vi "SEQUENCE_subVI_V2.vi"(0 "current step # in":i32, 5 "user sequence in":dbl[][](array[numeric]), 9 "input data":T1) -> (2 "pressure control settings out":T2, 3 "sequence on?":bool, 4 "vapor and gas flow out":dbl[](array[numeric]), 6 "sequence end time":timestamp, 10 "current  step # out":i32, 12 "time spent running":dbl)   [LabVIEW 2014]
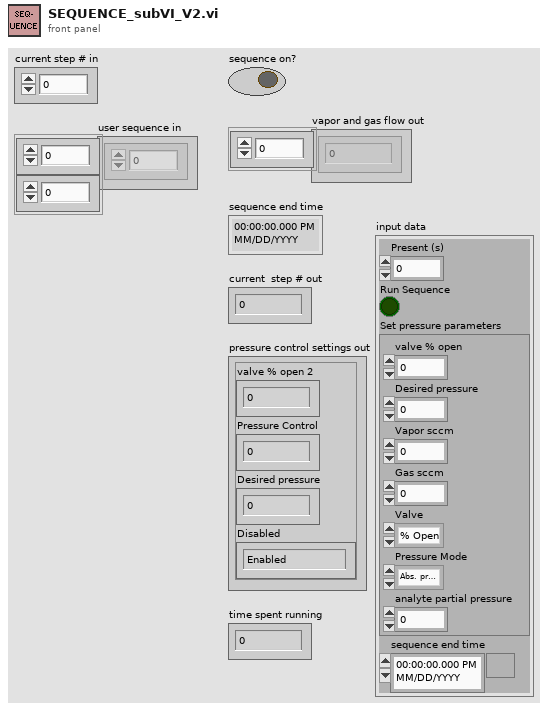
[diagram p1: front panel]
types:
  T1 = cluster{"Present (s)":dbl, "Run Sequence":bool, "Set pressure parameters":cluster{"valve % open":dbl, "Desired pressure":dbl, "Vapor sccm":sgl, "Gas sccm":sgl, "Valve":enum32{"% Open", "Torr "}, "Pressure Mode":enum32{"Abs. pressure", " Part. pressure"}, "analyte partial pressure":dbl}, "sequence end time":timestamp}
  T2 = cluster{"valve % open 2":dbl, "Pressure Control":u32, "Desired pressure":dbl, "Disabled":enum8{"Enabled", "Disabled", "Disabled and Grayed Out"}}
  T3 = cluster{"valve % open":dbl, "Desired pressure":dbl, "Vapor sccm":sgl, "Gas sccm":sgl, "Valve":enum32{"% Open", "Torr "}, "Pressure Mode":enum32{"Abs. pressure", " Part. pressure"}, "analyte partial pressure":dbl}
  T4 = enum8{"Enabled", "Disabled", "Disabled and Grayed Out"}
  T5 = cluster{"valve % open 2":dbl, "Pressure Control":u32, "Numeric Control":dbl, "Disabled":enum8{"Enabled", "Disabled", "Disabled and Grayed Out"}}
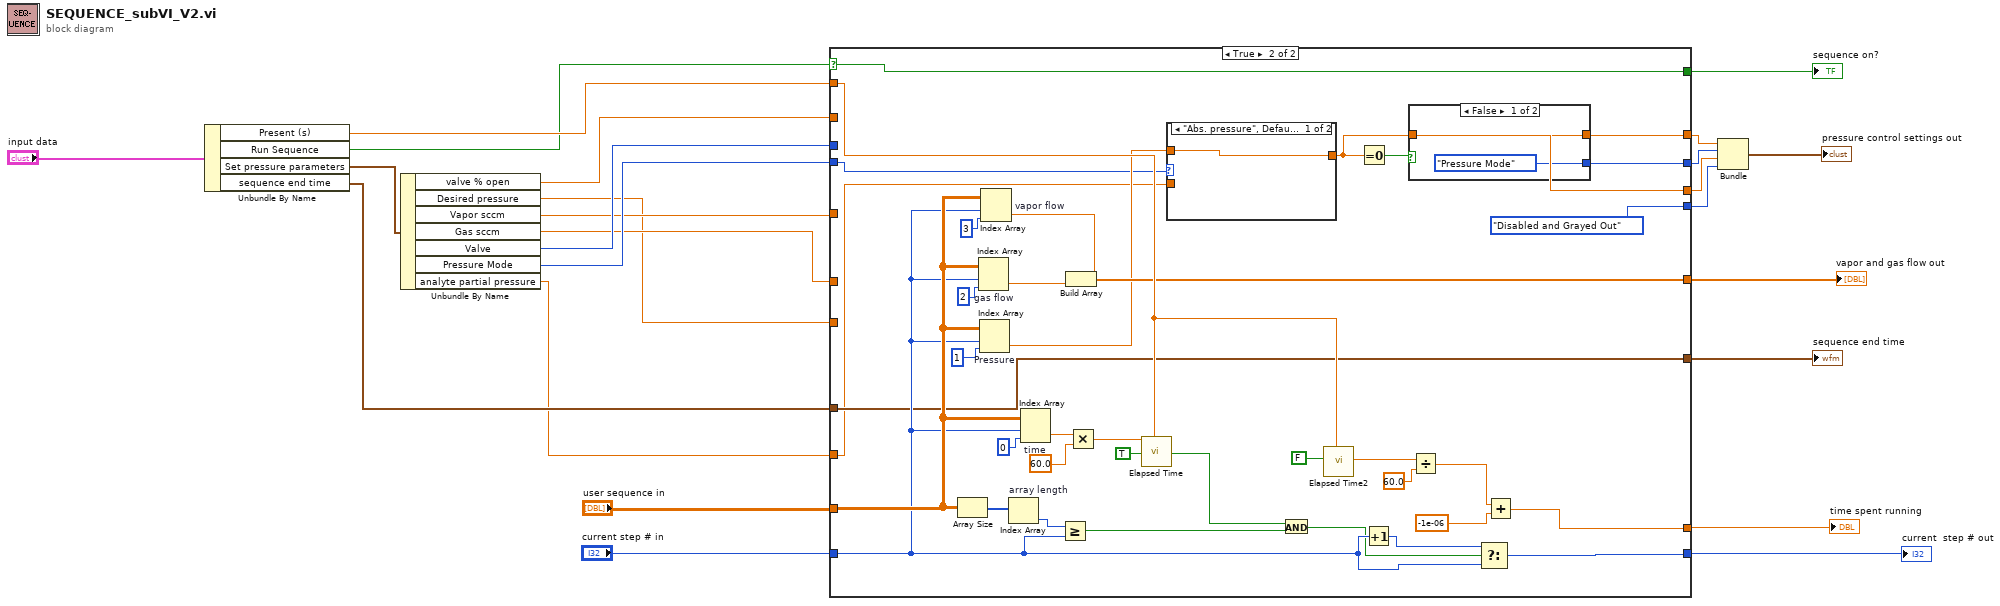
[diagram p0: block diagram]
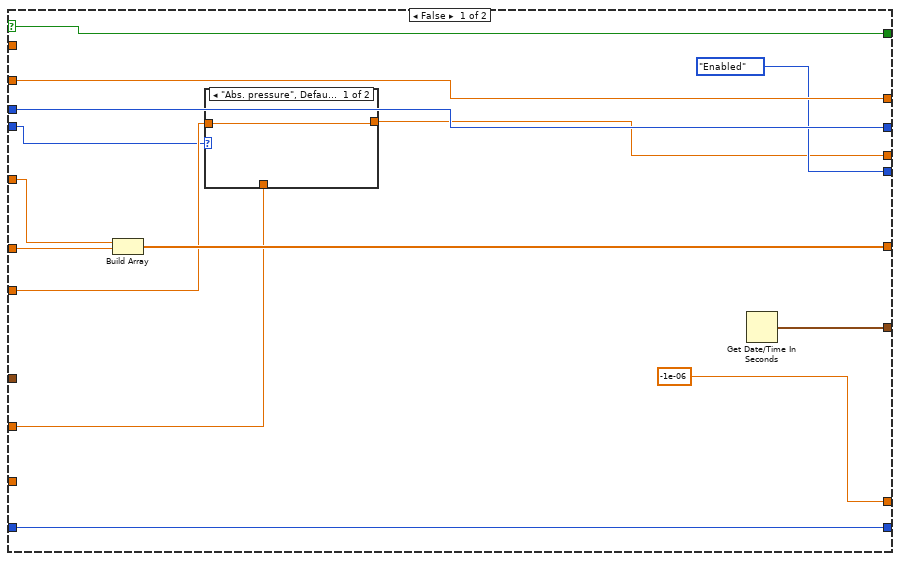
[diagram p2: hidden frame]
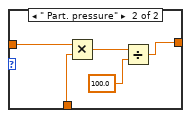
[diagram p3: hidden frame]
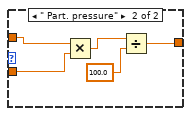
[diagram p4: hidden frame]
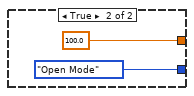
[diagram p5: hidden frame]
diagram:
  n1 = Unbundle By Name("input data") -> ("Present (s)"=w4:dbl, "Run Sequence"=w2:bool, "Set pressure parameters"=w3:T3, "sequence end time"=w12:timestamp)
  n2 = Unbundle By Name(w3) -> ("valve % open"=w10:dbl, "Desired pressure"=w5:dbl, "Vapor sccm"=w7:sgl, "Gas sccm"=w6:sgl, "Valve"=w9:enum32{"% Open", "Torr "}, "Pressure Mode"=w8:enum32{"Abs. pressure", " Part. pressure"}, "analyte partial pressure"=w11:dbl)
  n3 = case "Sequence" shown="True" w2 {
    selector: w2 -> [w35 w62]
    tunnel: w4 -> [_ w70]
    tunnel: [w38 w71] -> w13
    tunnel: "current step # in" -> [w38 w63]
    tunnel: w7 -> [w33 _]
    tunnel: w6 -> [w32 _]
    tunnel: [w28 w48] -> w20
    tunnel: "user sequence in" -> [_ w65]
    tunnel: w9 -> [w37 _]
    tunnel: [w37 w58] -> w19
    tunnel: [-1e-06 w50] -> w15
    tunnel: [w35 w62] -> w16
    tunnel: [w34 w59] -> w22
    tunnel: w10 -> [w34 _]
    tunnel: [w31 w55] -> w24
    tunnel: [T4."Enabled" ("Disabled") T4."Disabled and Grayed Out" ("Disabled")] -> w23
    tunnel: [w29 w53] -> w17
    tunnel: w12 -> [_ w53]
    tunnel: w5 -> [w27 _]
    tunnel: w11 -> [w26 w47]
    tunnel: w8 -> [w25 w46]
    frame False {
      n4 = Build Array(w33, w32) -> (w31:sgl[])
      n5 = case shown="\"Abs. pressure\", Default" w25 {
        tunnel: [w39 w40] -> w28
        tunnel: w27 -> [w39 w42]
        tunnel: w26 -> [_ w41]
        frame "Abs. pressure", Default {
        }
        frame " Part. pressure" {
          n6 = Multiply(x=w42, y=w41) -> (x*y=w44:dbl)
          n7 = Divide(x=w44, y=100.0 ("Analyte part. press. (%)")) -> (x/y=w40:dbl)
        }
      }
      n8 = Get Date/Time In Seconds() -> (seconds since 1Jan1904=w29:timestamp)
    }
    frame True {
      n9 = Array Size(array=w65) -> (size(s)=w81:i32[])
      n10 = Index Array "gas flow"(array=w65, index (row)=w63, index (col)=2 ("disabled index (col)")) -> (element=w56:dbl)
      n11 = Index Array "Pressure"(array=w65, index (row)=w63, index (col)=1 ("disabled index (col)")) -> (element=w49:dbl)
      n12 = Index Array "vapor flow"(array=w65, index (row)=w63, index (col)=3 ("disabled index (col)")) -> (element=w57:dbl)
      n13 = Index Array "array length"(array=w81) -> (element=w66:i32)  [unwired: 1 in]
      n14 = Index Array "time"(array=w65, index (row)=w63, index (col)=0) -> (element=w74:dbl)
      n15 = Greater Or Equal?(x=w66, y=w63) -> (x >= y?=w78:bool)
      n16 = Build Array(w57, w56) -> (w55:dbl[])
      n17 = Multiply(x=w74, y=60.0) -> (x*y=w64:dbl)
      n18 = call "Elapsed Time"("Time Target (s)"=w64, "Auto Reset"=TRUE, "Set Start Time (s)"=w70) -> ("Time has Elapsed"=w45:bool)  [unwired: 9 in, 7 out]
      n19 = case shown="\"Abs. pressure\", Default" w46 {
        tunnel: [w82 w83] -> w48
        tunnel: w49 -> [w82 w85]
        tunnel: w47 -> [_ w84]
        frame "Abs. pressure", Default {
        }
        frame " Part. pressure" {
          n20 = Multiply(x=w85, y=w84) -> (x*y=w86:dbl)
          n21 = Divide(x=w86, y=100.0 ("Analyte part. press. (%)")) -> (x/y=w83:dbl)
        }
      }
      n22 = And(x=w45, y=w78) -> (x .and. y?=w61:bool)
      n23 = call "Elapsed Time2"("Reset"=FALSE, "Set Start Time (s)"=w70) -> ("Elapsed Time (s)"=w68:dbl)  [unwired: 10 in, 7 out]
      n24 = Equal To 0?(x=w48) -> (x = 0?=w60:bool)
      n25 = Increment(x=w63) -> (x+1=w72:i32)
      n26 = case shown="False" w60 {
        tunnel: [enum32{"Open Mode", "Pressure Mode"}."Pressure Mode" ("Pressure Control") enum32{"Open Mode", "Pressure Mode"}."Open Mode" ("Pressure Control")] -> w58
        tunnel: [w88 100.0 ("valve % open 2")] -> w59
        tunnel: w48 -> [w88 _]
        frame False {
        }
        frame True {
        }
      }
      n27 = Divide(x=w68, y=60.0) -> (x/y=w52:dbl)
      n28 = Select(t=w72, s=w61, f=w63) -> (s? t:f=w71:i32)
      n29 = Add(x=w52, y=-1e-06) -> (x+y=w50:dbl)
    }
  }
  "vapor and gas flow out" <- w24
  "sequence end time" <- w17
  "sequence on?" <- w16
  "time spent running" <- w15
  "current  step # out" <- w13
  n30 = Bundle("valve % open 2"=w22, "Pressure Control"=w19, "Numeric Control"=w20, "Disabled"=w23) -> (→"pressure control settings out":T5)  [unwired: 1 in]
